vi "Untitled 1.vi"() -> ()   [LabVIEW 2017]
uses:
  <userlib>/Circular Buffer/Circular Buffer.lvlib
  <userlib>/Circular Buffer/Instance VIs/Circular Buffer(2D DBL).vi
panel:
  out "XY Graph":cluster{"Y":dbl[], "Y":dbl[]}[](graph)
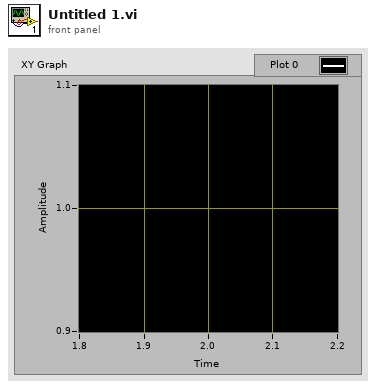
[diagram p1: front panel]
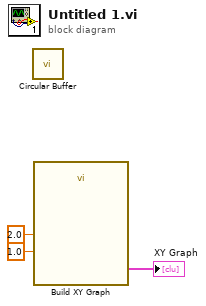
[diagram p0: block diagram]
diagram:
  n1 = call-poly <userlib>:"Circular Buffer.vi"() -> ()  [unwired: 8 in, 4 out]
  n2 = call "Build XY Graph"("Y Input"=1.0, "X Input"=2.0) -> ("XY Graph"=→"XY Graph":cluster{"X":dbl[], "Y":dbl[]}[])  [unwired: 8 in, 1 out]
